vi "SineGlobals.vi"() -> ()   [LabVIEW 2019]
panel:
  out "Time Constant":dbl
  out "Freq":dbl
  out "PeakAmp":dbl
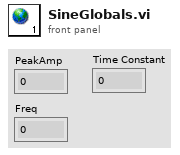
[diagram p1: front panel]
diagram:
